vi "WriteHeader.vi"(8 "error in (no error)":errorcluster, 10 "header":T1={"msg_id"="", "username"="", "session"="", "date"=timestamp(0 s since 1904-01-01), "msg_type"="", "version"="5.0"}, 11 "object in":refnum<class "Message Class.lvclass">) -> (0 "error out":errorcluster, 3 "object out":refnum<class "Message Class.lvclass">)   [LabVIEW 2018, in "ClientMessaging.lvlib" / "Message Class.lvclass"]
uses:
  Message Class.lvclass
  protected/header_dict.ctl
  Message Class.lvclass/Message Class.ctl
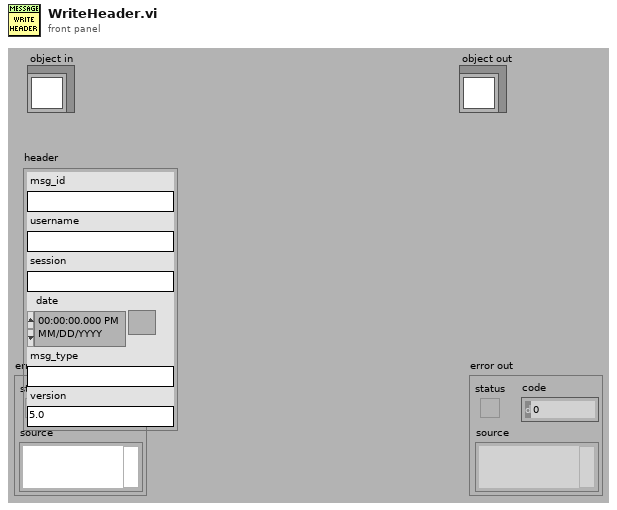
[diagram p1: front panel]
types:
  T1 = typedef "ClientMessaging.lvlib/Message Class.lvclass/header_dict.ctl" = cluster{"msg_id":string, "username":string, "session":string, "date":timestamp, "msg_type":string, "version":string}
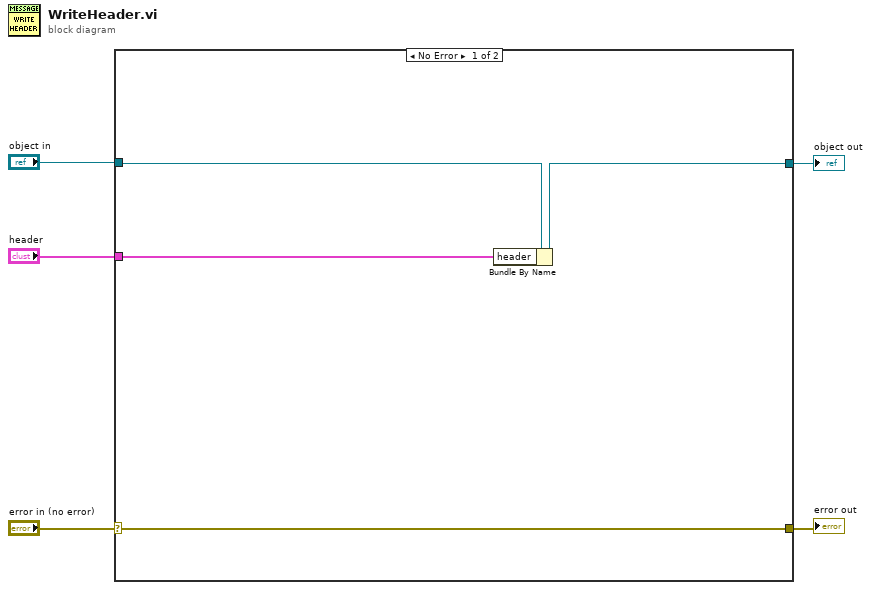
[diagram p0: block diagram]
diagram:
  n1 = case shown="No Error" "error in (no error)" {
    selector: "error in (no error)" -> [w8 w11]
    tunnel: [w8 w11] -> w4
    tunnel: [w6 w10] -> w2
    tunnel: "object in" -> [w7 w10]
    tunnel: "header" -> [w9 _]
    frame No Error {
      n2 = Bundle By Name(cluster=w7, "header"=w9) -> (w6:refnum<class "Message Class.lvclass">)
    }
    frame Error {
    }
  }
  "error out" <- w4
  "object out" <- w2
